vi "Query Trace Data.vi"(8 "error in (no error)":errorcluster, 10 "Trace Number":u8=1, 11 "VNA-Ag87xx in":refnum<class "VNA-Ag87xx.lvclass">) -> (0 "error out":errorcluster, 1 "Data":dbl[](array[numeric]), 2 "Frequency":dbl[](array[numeric]), 3 "VNA-Ag87xx out":refnum<class "VNA-Ag87xx.lvclass">)   [LabVIEW 2020, in "VNA-Ag87xx.lvclass"]
doc: "Query the active trace data.\nIt returns both x and y data"
uses:
  VNA-Ag87xx.lvclass
  C:/Sandbox/RF Bench/Source Code/WiSpry Test Framework/Instruments/Instrument.lvclass
  Instrument.lvclass/Instrument.ctl
  Instrument.lvclass
  <instrlib>/Agilent 87XX Series/Agilent 87XX Series.lvlib
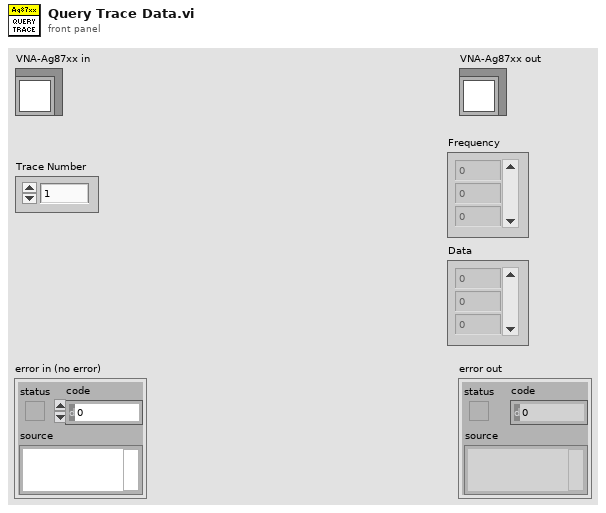
[diagram p1: front panel]
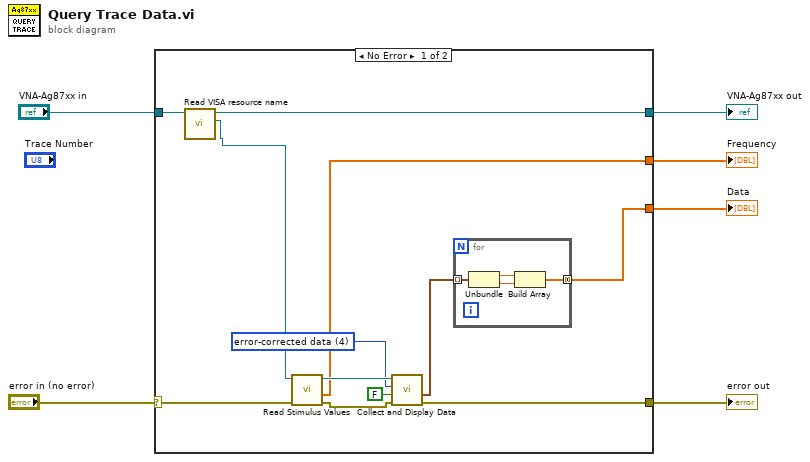
[diagram p0: block diagram]
diagram:
  n1 = case shown="No Error" "error in (no error)" {
    selector: "error in (no error)" -> [w9 w23]
    tunnel: [w17 w24] -> w4
    tunnel: "VNA-Ag87xx in" -> [w18 w24]
    tunnel: [w8 w23] -> w5
    tunnel: [w14 _] -> w2
    tunnel: [w10 _] -> w1
    frame No Error {
      w12 = u16 4 items=["raw data array 1", "raw data array 2", "raw data array 3", "raw data array 4", "error-corrected data", "error-corrected trace memory", "formatted data", "formatted memory", "formatted data / memory", "formatted data - memory"] ("data type (6 : formatted data)")
      n2 = call "Read VISA resource name.vi"("Instrument in"=w18) -> ("VISA resource name"=w15:refnum<visa-resource-name>, "Instrument out"=w17:refnum<class "VNA-Ag87xx.lvclass">)  [unwired: 9 in]
      n3 = call <instrlib>:"Read Stimulus Values.vi"("error in (no error)"=w9, "VISA resource name"=w15) -> ("error out"=w7:errorcluster, "stimulus list"=w14:dbl[], "VISA resource name out"=w16:refnum<visa-resource-name>)  [unwired: 7 in]
      n4 = call <instrlib>:"Collect and Display Data.vi"("error in (no error)"=w7, "save to file"=FALSE, "data type (6 : formatted data)"=w12, "VISA resource name"=w16) -> ("error out"=w8:errorcluster, "data values"=w11:cluster{"real / stim":dbl, "imag / resp":sgl}[])  [unwired: 4 in, 2 out]
      n5 = for {
        tunnel: w11 -> [w22] mode=indexing
        tunnel: [w19] -> w10 mode=concatenating
        n6 = Unbundle(w22) -> ("real / stim"=w21:dbl, "imag / resp"=w20:sgl)
        n7 = Build Array(w21, w20) -> (w19:dbl[])
      }
    }
    frame Error {
    }
  }
  "error out" <- w5
  "VNA-Ag87xx out" <- w4
  "Data" <- w1
  "Frequency" <- w2
